vi "permissions_set-icacls.vi"(8 "error in (no error)":errorcluster, 9 "simple_permission":T1, 10 "group_user":string, 11 "filepath in":path) -> (0 "error out":errorcluster, 3 "filepath out":path)   [LabVIEW 2015, in "lv-bin-windows.lvlib" / "v1.lvlib"]
uses:
  v1.lvlib
  _controls/permission.ctl
  <userlib>/antonio-alexander/lv-bin/lv-bin/public/api/v1/v1.lvlib
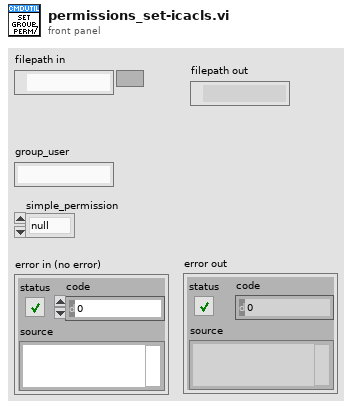
[diagram p1: front panel]
types:
  T1 = typedef "lv-bin-windows.lvlib/v1.lvlib/permission.ctl" = enum16{"null", "none n", "full f", "modify m", "read_execute rx", "read_only r", "write_only w", "delete d"}
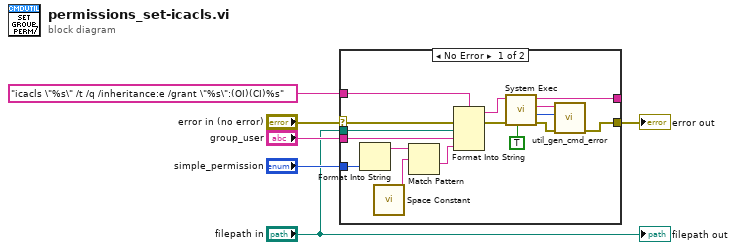
[diagram p0: block diagram]
diagram:
  n1 = case shown="No Error" "error in (no error)" {
    selector: "error in (no error)" -> [w18 w23]
    tunnel: "simple_permission" -> [w22 _]
    tunnel: "icacls \"%s\" /t /q /inheritance:e /grant \"%s\":(OI)(CI)%s" -> [w19 _]
    tunnel: "group_user" -> [w17 _]
    tunnel: [w11 w23] -> w2
    tunnel: "filepath in" -> [w10 _]
    tunnel: [w9 _] -> _
    frame No Error {
      n2 = Format Into String(w22) -> (resulting string=w21:string)  [unwired: 3 in, 1 out]
      n3 = call <vilib>:"Space Constant.vi"() -> ("String"=w20:string)
      n4 = Match Pattern(string=w21, regular expression=w20) -> (after substring=w16:string)  [unwired: 1 in, 3 out]
      n5 = Format Into String(format string=w19, error in=w18, w10, w17, w16) -> (resulting string=w14:string, error out=w15:errorcluster)  [unwired: 1 in]
      n6 = call <vilib>:"System Exec.vi"("run minimized? (F)"=TRUE, "error in (no error)"=w15, "command line"=w14) -> ("error out"=w12:errorcluster, "return code"=w7:i32, "standard error"=w8:string, "standard output"=w9:string)  [unwired: 5 in]
      n7 = call <userlib>:"util_gen_cmd_error.vi"("error in (no error)"=w12, "return_code"=w7, "standard_error"=w8) -> ("error out"=w11:errorcluster)  [unwired: 8 in]
    }
    frame Error {
    }
  }
  "error out" <- w2
  "filepath out" <- "filepath in"
